vi "SR430.Set Trigger Offset us.vi"(0 "i ref in":refnum<vi>, 7 "triggerOffset [us]":i32, 11 "error in (no error)":errorcluster) -> (4 "i ref out":refnum<vi>, 15 "error out":errorcluster)   [LabVIEW 2014, in "SR430.lvlib"]
doc: "by Romain Savreux"
uses:
  SR430.lvlib
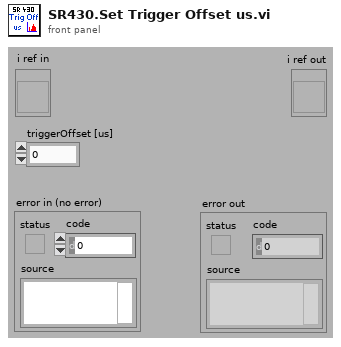
[diagram p1: front panel]
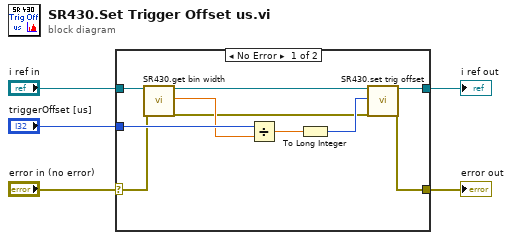
[diagram p0: block diagram]
diagram:
  n1 = case shown="No Error" "error in (no error)" {
    selector: "error in (no error)" -> [w6 w16]
    tunnel: "triggerOffset [us]" -> [w15 _]
    tunnel: [w10 w16] -> w4
    tunnel: [w9 w17] -> w3
    tunnel: "i ref in" -> [w7 w17]
    frame No Error {
      n2 = call "SR430.get bin width.vi"("i ref in"=w7, "error in (no error)"=w6) -> ("i ref out"=w8:refnum<vi>, "binWidth [us]"=w14:dbl, "error out"=w11:errorcluster)  [unwired: 15 in]
      n3 = Divide(x=w15, y=w14) -> (x/y=w13:dbl)
      n4 = To Long Integer(number=w13) -> (32bit integer=w12:i32)
      n5 = call "SR430.set trig offset.vi"("i ref in"=w8, "triggerOffset"=w12, "error in (no error)"=w11) -> ("i ref out"=w9:refnum<vi>, "error out"=w10:errorcluster)  [unwired: 14 in, 1 out]
    }
    frame Error {
    }
  }
  "error out" <- w4
  "i ref out" <- w3
